vi "Multirate Filtering.vi"() -> ()   [LabVIEW 2023]
doc: "Demonstrates how to use the DFD MRate Filtering for Single Block VI to filter a signal and how to perform a zero-phase multirate filtering.\n\nComplete the following steps to use this VI.\n1) Run the VI.\n2) Change the <B>Filtering Mode</B>, run the VI again, and observe the number of samples in the Signal Out plot.\n3) Set the <B>Zero Phase?</B> value to off (FALSE), run the VI again, and observe the delay between the Signal In and Signal Out plots.\n4) Change the <B>Extension Type</B> option, run the VI again, and zoom in the Signals graph to observe the effect on the filtered signal."
uses:
  <vilib>/addons/Digital Filter Design/_Objects.llb/DFD Multirate Filtering Mode.ctl
  <vilib>/addons/Digital Filter Design/_Objects.llb/DFD Multirate Filter Specification (Design).ctl
  <vilib>/addons/Digital Filter Design/_Objects.llb/DFD Filter Ripple Specification (Design).ctl
  <vilib>/addons/Digital Filter Design/Design.llb/DFD MRate Filter Design (Integer).vi
  <vilib>/addons/Digital Filter Design/Multirate.llb/DFD MRate Filtering for Single Block (Wfm).vi
  <vilib>/measure/NI_MABase.lvlib
  <vilib>/addons/Digital Filter Design/NI_DigFilterLicensed.lvlib
panel:
  out "Error Message":string
  in  "Extension Type":u16(ring) items=["Zero padding", "Symmetric", "Periodic"]
  in  "Filtering Mode":T1=2 items=["No Rate Change", "Interpolation", "Decimation"]
  out "Signals":waveform(dbl)[](graph)=[{"t0"=timestamp(0 s since 1904-01-01), "dt"=1.0, "Y"=[]}, {"t0"=timestamp(0 s since 1904-01-01), "dt"=1.0, "Y"=[]}]
  in  "Zero Phase?":bool=TRUE
  # "Select Help>>Show Context Help and move the cursor over the VI icon for more information."
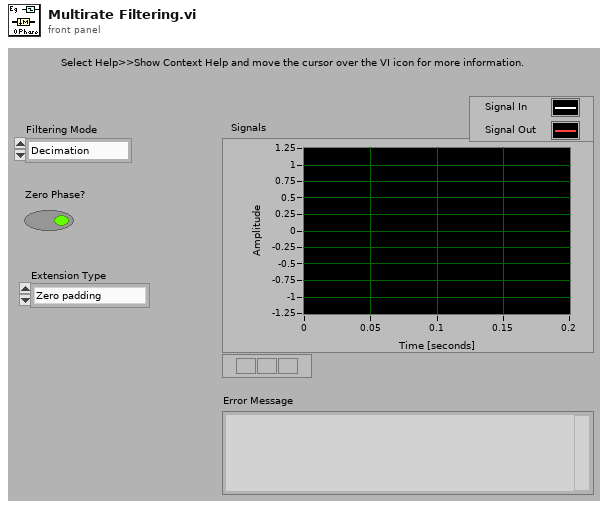
[diagram p1: front panel]
types:
  T1 = typedef "NI_DigFilterLicensed.lvlib/DFD Multirate Filtering Mode.ctl" = u16
  T2 = typedef "NI_DigFilterLicensed.lvlib/DFD Filter Ripple Specification (Design).ctl" = cluster{"passband":dbl, "stopband":dbl, "dB/linear? (T: dB)":bool}
  T3 = typedef "NI_DigFilterLicensed.lvlib/DFD Multirate Filter Specification (Design).ctl" = cluster{"fpass":dbl, "fstop":dbl}
  T4 = typedef "NI_DigFilterLicensed.lvlib/DFD Multirate Filter Obj.ctl" = cluster{"mMRate_Structure":enum16{"CIC", "FIR", "IIR", "Lattice"}, "mMRate_Mode":T5, "mMRate_Factor":i32, "mMRate_FIRParams":cluster{"mMRate_FIR_H":dbl[], "mMRate_FIR_IsNyquist?":bool, "mMRate_FIR_IsSymmetric?":bool}, "mMRate_CICParams":cluster{"mMRate_CIC_#Stage":i32, "mMRate_CIC_Lag":i32, "mMRate_CIC_Type":enum16{"Lowpass", "Highpass"}}, "mMRate_Order":i32, "mMRate_Version":string, "mMRate_Comments":string, "mMRate_RationalFactor":cluster{"mMRate_L":i32, "mMRate_M":i32}, "mMRate_Fs":dbl, "mMRate_Quantized?":bool, "mMRate_QFilterGain":dbl, "mMRate_CoefWl":i16, "mMRate_Scaling":cluster{"mMRate_ScaleByPowerOf2?":bool, "mMRate_ScaleType":T6}, "mMRate_InputWl":i16, "mMRate_OutputWl":i16, "mMRate_OutputMode":T7, "mMRate_MultMode":T8, "mMRate_BitPruning":bool, "mMRate_GainWl":i16, "mMRate_OutputFwl":i16, "mMRate_SumIwl":i16, "mMRate_InputIwl ":i16, "mMRate_SumWl":i16, "mMRate_CoefIwl":i16}
  T5 = typedef "NI_DigFilterLicensed.lvlib/DFD Multirate Mode.ctl" = i16
  T6 = typedef "NI_DigFilterLicensed.lvlib/DFD Coef Norm Type.ctl" = enum16{"No Norm", "Time Domain 1-Norm", "Time Domain 2-Norm", "Time Domain Inf-Norm"}
  T7 = typedef "NI_DigFilterLicensed.lvlib/DFD Round-off Mode.ctl" = enum16{"Nearest", "Truncation"}
  T8 = typedef "NI_DigFilterLicensed.lvlib/DFD FXP MRate Multiply Mode.ctl" = enum16{"Truncated", "Full"}
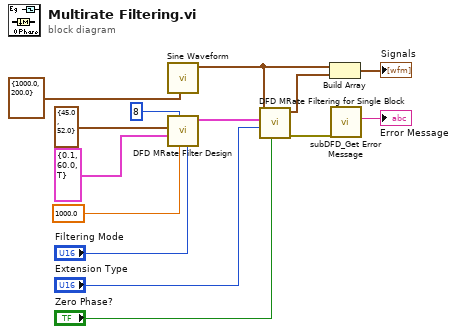
[diagram p0: block diagram]
diagram:
  n1 = call <vilib>:"Sine Waveform.vi"("sampling info"=cluster{"Fs":dbl, "#s":dbl} {"Fs"=1000.0, "#s"=200.0}) -> ("signal out"=w10:waveform(dbl))  [unwired: 6 in, 4 out]
  n2 = call-poly <vilib>:"DFD MRate Filter Design.vi"("filtering mode"="Filtering Mode", "fs in [Hz]"=1000.0 ("fs [Hz]"), "factor"=8 ("multirate factor"), "ripple specs"=T2 {"passband"=0.1, "stopband"=60.0, "dB/linear? (T: dB)"=TRUE}, "freq specs [Hz]"=T3 {"fpass"=45.0, "fstop"=52.0}) -> ("multirate filter out"=w11:T4)  [unwired: 3 in, 3 out]
  n3 = call-poly <vilib>:"DFD MRate Filtering for Single Block.vi"("zero phase? (T)"="Zero Phase?", "extension type"="Extension Type", "multirate filter"=w11, "signal in"=w10) -> ("error out"=w1:errorcluster, "signal out"=w14:waveform(dbl))  [unwired: 1 in, 5 out]
  n4 = Build Array(w10, w14) -> (→"Signals":waveform(dbl)[])
  n5 = call <vilib>:"subDFD_Get Error Message.vi"("error in (no error)"=w1) -> ("Error Message"=→"Error Message":string)  [unwired: 10 out]
